vi "Import QD ShortCut.vi"() -> ()   [LabVIEW 2014]
uses:
  <resource>/dialog/lvconfig.llb/LV Config Read String.vi
  <vilib>/Utility/config.llb/Read Key (String).vi
  <vilib>/Utility/config.llb/NI_LVConfig.lvlib
panel:
  out "value":string
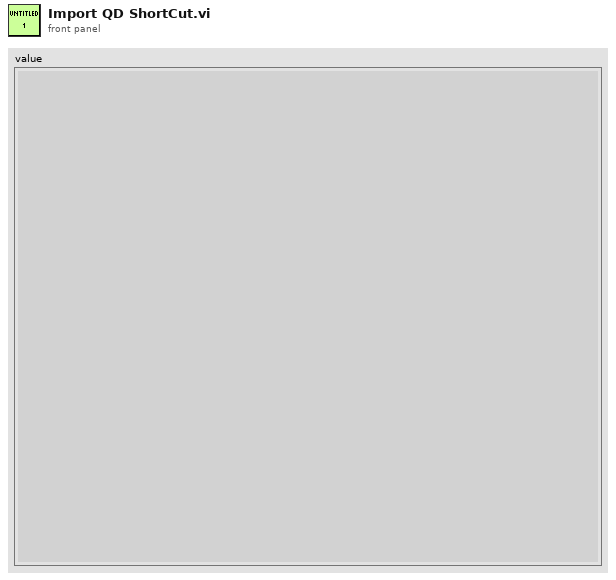
[diagram p1: front panel]
types:
  T1 = typedef "NI_LVConfig.lvlib/Config Data RefNum.ctl" = refnum<k1>
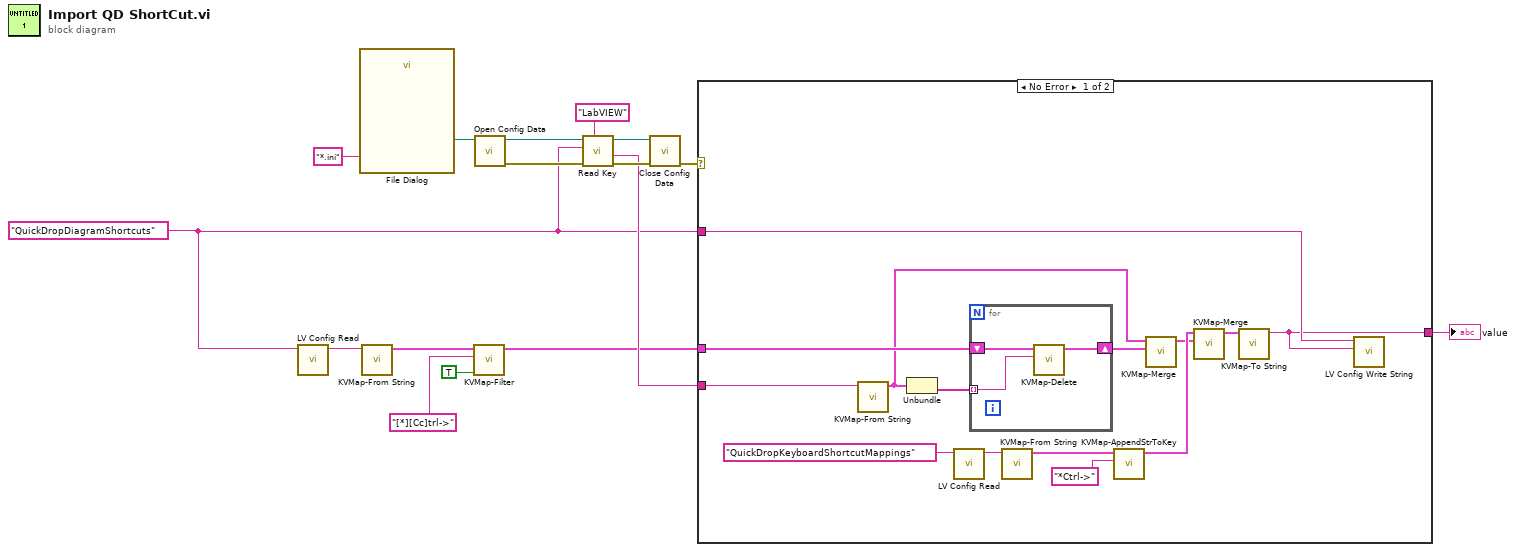
[diagram p0: block diagram]
diagram:
  w3 = "QuickDropDiagramShortcuts" ("key")
  n1 = call-poly <resource>:"LV Config Read.vi"("key"=w3) -> ("value"=w16:string)  [unwired: 4 in, 2 out]
  n2 = call "File Dialog"("pattern (all files)"="*.ini") -> ("selected path"=w12:path)  [unwired: 11 in, 3 out]
  n3 = call "KVMap-From String.vi"("value"=w16) -> ("Cluster"=w15:cluster{string[], string[]})  [unwired: 10 in]
  n4 = call "KVMap-Filter.vi"("T->First/F->Second(F)"=TRUE, "filter"="[*][Cc]trl->", "Cluster in"=w15) -> ("Cluster out"=w4:cluster{string[], string[]})  [unwired: 8 in]
  n5 = call <vilib>:"Open Config Data.vi"("configuration file path"=w12) -> ("error out"=w9:errorcluster, "refnum"=w11:T1)  [unwired: 8 in, 1 out]
  n6 = call-poly <vilib>:"Read Key.vi"("section"="LabVIEW", "error in (no error)"=w9, "key"=w3, "refnum"=w11) -> ("error out"=w8:errorcluster, "value"=w5:string, "refnum out"=w10:T1)  [unwired: 4 in, 1 out]
  n7 = call <vilib>:"Close Config Data.vi"("error in (no error)"=w8, "refnum"=w10) -> ("error out"=w1:errorcluster)  [unwired: 8 in, 1 out]
  n8 = case shown="No Error" w1 {
    tunnel: w5 -> [w30 _]
    tunnel: w4 -> [w27 _]
    tunnel: w3 -> [w18 _]
    tunnel: [w17 _] -> w2
    frame No Error {
      n9 = call "KVMap-From String.vi"("value"=w30) -> ("Cluster"=w26:cluster{string[], string[]})  [unwired: 10 in]
      n10 = Unbundle(w26) -> (w29:string[])  [unwired: 1 out]
      n11 = call-poly <resource>:"LV Config Read.vi"("key"="QuickDropKeyboardShortcutMappings") -> ("value"=w24:string)  [unwired: 4 in, 2 out]
      n12 = for {
        shift-right: [w32] -> w28
        shift-left: w27 -> [w33]
        tunnel: w29 -> [w31] mode=indexing
        n13 = call "KVMap-Delete.vi"("element"=w31, "Cluster in"=w33) -> ("Cluster out"=w32:cluster{string[], string[]})  [unwired: 9 in]
      }
      n14 = call "KVMap-From String.vi"("value"=w24) -> ("Cluster"=w22:cluster{string[], string[]})  [unwired: 10 in]
      n15 = call "KVMap-AppendStrToKey.vi"("string"="*Ctrl->", "Cluster in"=w22) -> ("Cluster out"=w21:cluster{string[], string[]})  [unwired: 9 in]
      n16 = call "KVMap-Merge.vi"("Cluster 2"=w28, "Cluster in"=w26) -> ("Cluster"=w19:cluster{string[], string[]})  [unwired: 8 in]
      n17 = call "KVMap-Merge.vi"("Cluster 2"=w19, "Cluster in"=w21) -> ("Cluster"=w20:cluster{string[], string[]})  [unwired: 8 in]
      n18 = call "KVMap-To String.vi"("Cluster"=w20) -> ("value"=w17:string)  [unwired: 10 in]
      n19 = call <resource>:"LV Config Write String.vi"("value"=w17, "key"=w18) -> ()  [unwired: 5 in, 1 out]
    }
    frame Error {
    }
  }
  "value" <- w2
